vi "Handle String Data.vi"(7 "Source ID":u32, 8 "StringData":T1, 9 "Sequence":u32, 10 "ChannelService":refnum<class "ChannelService.lvclass">, 11 "Subscription Loop Data in":T2) -> (0 "error out":errorcluster, 3 "Subscription Loop Data":T2)   [LabVIEW 2020, in "Vecto.lvlib" / "RemoteDataService.lvclass"]
uses:
  RemoteDataService.lvclass
  RemoteDataService.lvclass/RemoteDataService.ctl
  ChannelService/ChannelService.lvclass
  <vilib>/Utility/miscctls.llb/LVMapReplaceAction.ctl
  StringGroup/StringGroup.lvclass
  C:/dev/lv20CE/relink/lv-vecto/Vecto/GroupAbstract/GroupAbstract.lvclass
  C:/dev/lv20CE/relink/lv-vecto/Vecto/StringGroup/StringGroup.lvclass
  Subscription Group Info.ctl
  Subscription Loop Data.ctl
  proto/StringData/Data.ctl
  proto/StringData/StringData.lvlib
  GroupAbstract/GroupAbstract.lvclass
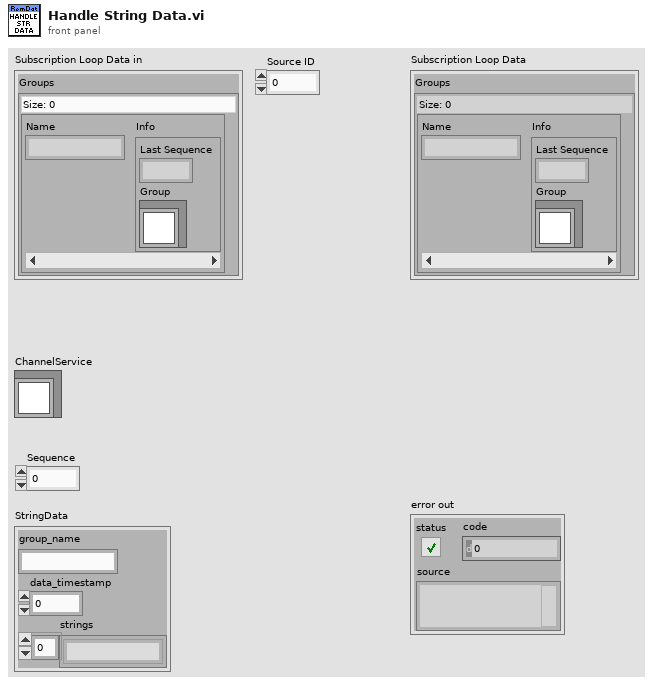
[diagram p1: front panel]
types:
  T1 = typedef "StringData.lvlib/Data.ctl" = cluster{"group_name":string, "data_timestamp":i64, "strings":string[]}
  T2 = typedef "Vecto.lvlib/RemoteDataService.lvclass/Subscription Loop Data.ctl" = cluster{"Groups":map{string, T3}}
  T3 = typedef "Vecto.lvlib/RemoteDataService.lvclass/Subscription Group Info.ctl" = cluster{"Last Sequence":u32, "Group":refnum<class "GroupAbstract.lvclass">}
  T4 = typedef "LVMapReplaceAction.ctl" = enum32{"Modify Entry only if found", "Add or Modify Entry", "Delete Entry"}
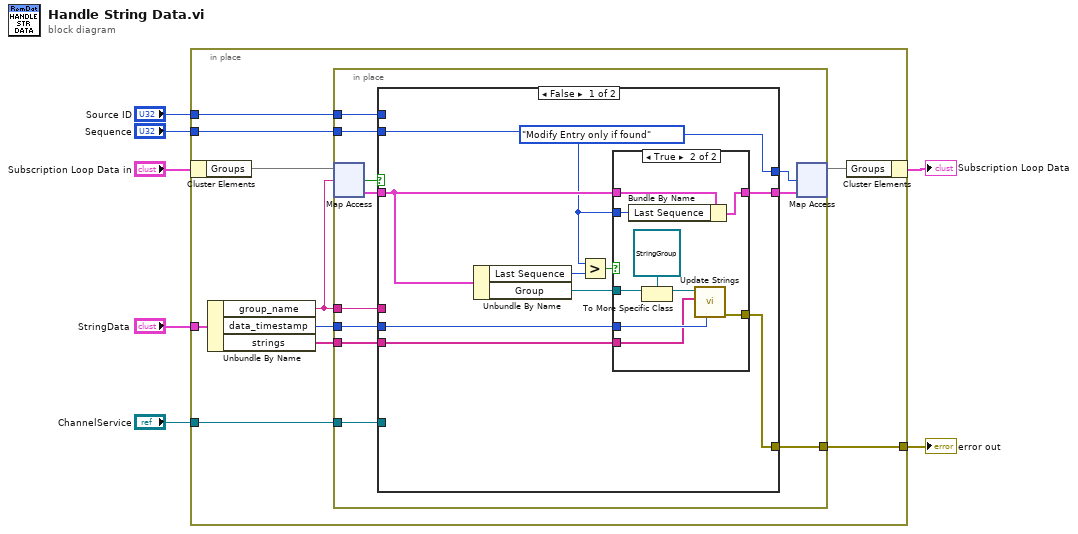
[diagram p0: block diagram]
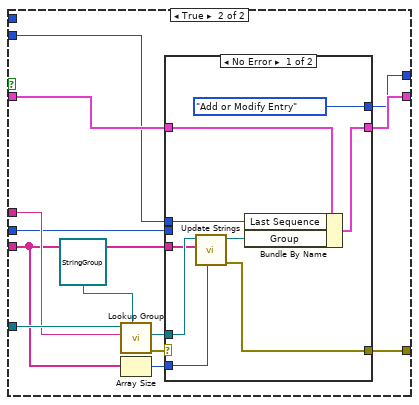
[diagram p3: hidden frame]
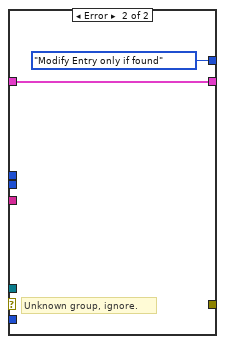
[diagram p4: hidden frame]
diagram:
  n1 = in-place {
    in-place-border: "StringData" -> [w8]
    in-place-border: "ChannelService" -> [w16]
    in-place-border: "Sequence" -> [w12]
    in-place-border: "Source ID" -> [w11]
    in-place-border: [w9] -> w2
    n2 = in-place-cluster #1("Subscription Loop Data in") -> ("Groups"=w17:map{string, T3})
    n3 = Unbundle By Name(w8) -> ("group_name"=w15:string, "data_timestamp"=w13:i64, "strings"=w14:string[])
    n4 = in-place {
      in-place-border: w16 -> [w26]
      in-place-border: w15 -> [w25]
      in-place-border: w14 -> [w24]
      in-place-border: w13 -> [w23]
      in-place-border: w12 -> [w22]
      in-place-border: w11 -> [w21]
      in-place-border: [w19] -> w9
      n5 = in-place-map #2(w17, w15) -> (w27:T3, w28:bool)  [unwired: 1 in]
      n6 = case shown="False" w28 {
        tunnel: w27 -> [w33 w56]
        tunnel: w26 -> [_ w61]
        tunnel: w25 -> [_ w59]
        tunnel: w24 -> [w34 w53]
        tunnel: w23 -> [w35 w54]
        tunnel: w22 -> [w31 w55]
        tunnel: w21 -> [_ _]
        tunnel: [w32 w52] -> w20
        tunnel: [w30 w51] -> w19
        tunnel: [LVMapReplaceAction."Modify Entry only if found" ("action") w50] -> w18
        frame False {
          n7 = Unbundle By Name(w33) -> ("Last Sequence"=w38:u32, "Group"=w37:refnum<class "GroupAbstract.lvclass">)
          n8 = Greater?(x=w31, y=w38) -> (0:w36:bool)
          n9 = case shown="True" w36 {
            tunnel: w37 -> [_ w48]
            tunnel: w35 -> [_ w47]
            tunnel: w34 -> [_ w40]
            tunnel: w33 -> [w39 w46]
            tunnel: [w39 w44] -> w32
            tunnel: w31 -> [_ w45]
            tunnel: [_ w43] -> w30
            frame False {
              # "Older data, ignore"
            }
            frame True {
              n10 = Bundle By Name(cluster=w46, "Last Sequence"=w45) -> (w44:T3)
              n11 = To More Specific Class(target class=refnum<class "StringGroup.lvclass"> refnum ("StringGroup in"), reference=w48) -> (specific class reference=w42:refnum<class "StringGroup.lvclass">)  [unwired: 1 in, 1 out]
              n12 = call "Update Strings.vi"("Timestamp (Now)"=w47, "Strings"=w40, "StringGroup in"=w42) -> ("error out"=w43:errorcluster)  [unwired: 7 in, 1 out]
            }
          }
        }
        frame True {
          n13 = call "Lookup Group.vi"("Group Type (Abstract)"=refnum<class "StringGroup.lvclass"> refnum ("Vecto.lvlib:StringGroup.lvclass"), "Group Name"=w59, "ChannelService in"=w61) -> ("error out"=w60:errorcluster, "Group"=w58:refnum<class "StringGroup.lvclass">)  [unwired: 6 in, 1 out]
          n14 = Array Size(array=w53) -> (size(s)=w57:i32)
          n15 = case shown="No Error" w60 {
            tunnel: w58 -> [w64 _]
            tunnel: w57 -> [w63 _]
            tunnel: w56 -> [w70 w71]
            tunnel: w55 -> [w69 _]
            tunnel: w54 -> [_ _]
            tunnel: w53 -> [w62 _]
            tunnel: [w68 w71] -> w52
            tunnel: [w67 _] -> w51
            tunnel: [LVMapReplaceAction."Add or Modify Entry" ("action") LVMapReplaceAction."Modify Entry only if found" ("action")] -> w50
            frame No Error {
              n16 = call "Update Strings.vi"("Timestamp (Now)"=w63, "Strings"=w62, "StringGroup in"=w64) -> ("error out"=w67:errorcluster, "StringGroup out"=w66:refnum<class "StringGroup.lvclass">)  [unwired: 7 in]
              n17 = Bundle By Name(cluster=w70, "Last Sequence"=w69, "Group"=w66) -> (w68:T3)
            }
            frame Error {
              # "Unknown group, ignore."
            }
          }
        }
      }
      n18 = in-place-map #2(w20, w18) -> (w10:map{string, T3})  [unwired: 2 out]
    }
    n19 = in-place-cluster #1("Groups"=w10) -> (→"Subscription Loop Data":T2)
  }
  "error out" <- w2
